vi "ExampleInstrument.UI.Create UI.vi"(8 "error in (no error)":errorcluster, 10 "Instrument in":refnum<class "Instrument.lvclass">, 11 "Example Instrument UI in":refnum<class "ExampleInstrument.UI.lvclass">) -> (0 "error out":errorcluster, 3 "Example Instrument UI out":refnum<class "ExampleInstrument.UI.lvclass">)   [LabVIEW 2016, in "ExampleInstrument.UI.lvclass"]
uses:
  ExampleInstrument.UI.lvclass
  C:/Program Files (x86)/National Instruments/LabVIEW 2016/vi.lib/JKI/JKI SMO/SMO/SMO.lvclass
  lvsrc/SMOs/Instrument/Instrument.lvclass
  ExampleInstrument.UI.lvclass/ExampleInstrument.UI.ctl
  <vilib>/JKI/JKI SMO/SMO/SMO.lvclass
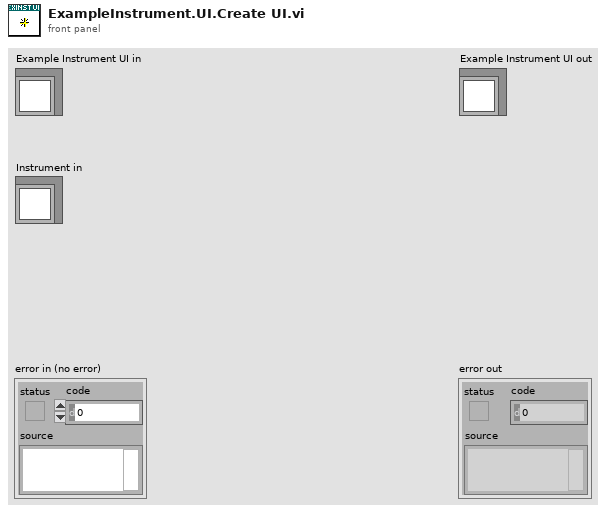
[diagram p1: front panel]
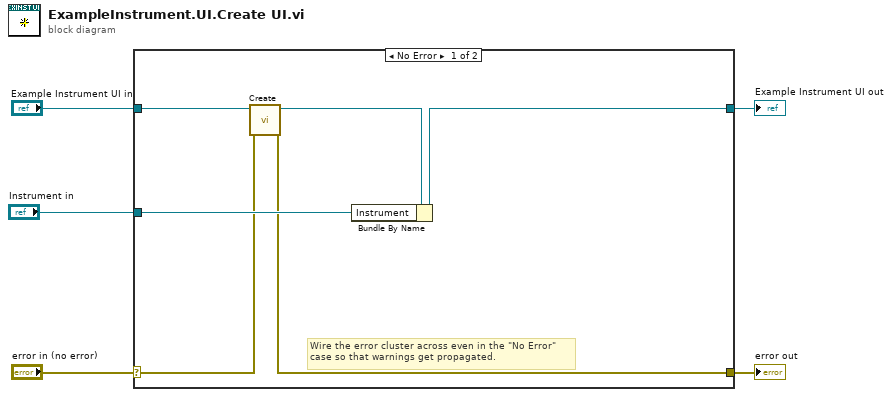
[diagram p0: block diagram]
diagram:
  n1 = case shown="No Error" "error in (no error)" {
    selector: "error in (no error)" -> [w7 w13]
    tunnel: [w6 w13] -> w4
    tunnel: [w11 w12] -> w2
    tunnel: "Example Instrument UI in" -> [w9 w12]
    tunnel: "Instrument in" -> [w10 _]
    frame No Error {
      # "Wire the error cluster across even in the \"No Error\"\ncase so that warnings get propagated."
      n2 = call <vilib>:"Create.vi"("error in (no error)"=w7, "SMO"=w9) -> ("error out"=w6:errorcluster, "SMO out"=w8:refnum<class "ExampleInstrument.UI.lvclass">)  [unwired: 7 in, 1 out]
      n3 = Bundle By Name(cluster=w8, "Instrument"=w10) -> (w11:refnum<class "ExampleInstrument.UI.lvclass">)
    }
    frame Error {
    }
  }
  "error out" <- w4
  "Example Instrument UI out" <- w2
